vi "ExPhotometricsAsync.vi"() -> ()   [LabVIEW 2010]
panel:
  in  "Shutter end state":u32(ring)=1 items=["N/A", "No Change (keep cc and shutter as is)", "Halt (No Cont Clears)", "Halt Close shutter (No cont. clears)", "Clear (turn on cont clears)", "Clear and close shutter (cc on, shutter closed)", "Open shutter (no cont clears)", "Clear and open shutter (cc on, shutter open)", ""]
  in  "Shutter State":u32(ring)=1 items=["N/A", "Shutter always closed.", "Shutter Normal (open for expos/close for readout)", "Shutter opened begin acquisition sequence", "Shutter open prior-trigger"]
  in  "Trigger Edge":u32(ring)=1 items=["N/A", "Positive (leading) edge", "Negative (falling) edge"]
  in  "Timing Mode":u32(ring)=1
  in  "Exposure":dbl min=0.0 step=0.001 format="%.3f"
  in  "stop":bool
  in  "Store":bool
  out "error out":errorcluster
  in  "error in (no error)":errorcluster
  # "ExPhotometricsAsync:\nThis is a Full Frame Async example dessigned specificly for \nPhotometrics cameras. This should work with \nall camera systems. It requires a start for every frame \ncollected. Not all timing modes work for all cameras, also \nthe trigger edge only applies to Princeton Instrument \ncameras. Not all cameras have the ability to set the \ntemperature.\nPressing the stop button stops the example."
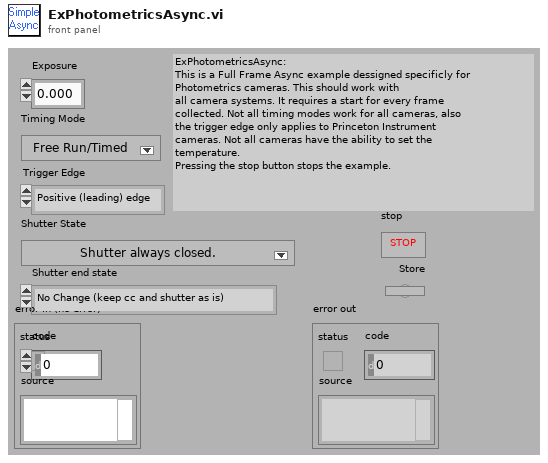
[diagram p1: front panel]
types:
  T1 = cluster{"Acquire mode \n3 is Async":i32, "Exposure":dbl, "Number of Images":i32, "Software Accums":i32}
  T2 = cluster{"Camera Handle":u32, "Pulser Handle":u32, "File Handle":u32, "Display Handle":u32, "Image Handle":u32}
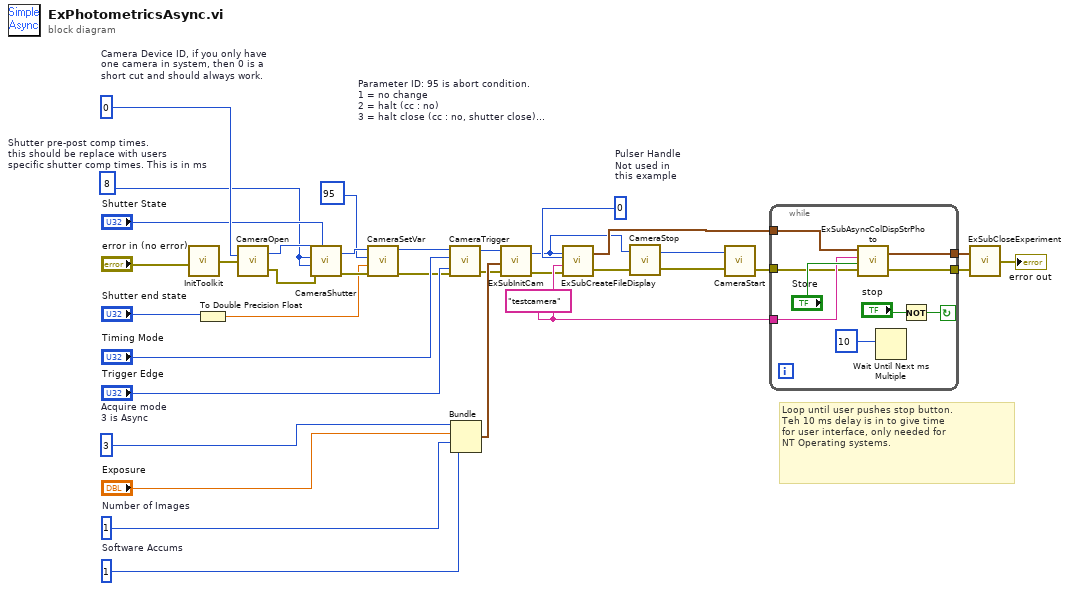
[diagram p0: block diagram]
diagram:
  w8 = 95  # Parameter ID: 95 is abort condition. 1 = no change 2 = halt (cc : no) 3 = halt close (cc : no, shutter close) 4 = clear (cc : yes) 5 = clear close (cc : yes, shutter close) 6 = open (cc : no, shutter open) 7 = clear open (cc : yes, shutter open)
  w13 = 8  # Shutter pre-post comp times. this should be replace with users  specific shutter comp times. This is in ms
  w21 = 0  # Camera Device ID, if you only have  one camera in system, then 0 is a  short cut and should always work.
  w28 = 0  # Pulser Handle Not used in  this example
  w33 = 1  # Number of Images
  w34 = 3  # Acquire mode  3 is Async
  w32 = 1  # Software Accums
  w35 = "testcamera"
  # "Loop until user pushes stop button.\nTeh 10 ms delay is in to give time \nfor user interface, only needed for \nNT Operating systems."
  n1 = call <userlib>:"InitToolkit.vi"("error in"="error in (no error)") -> ("error out"=w22:errorcluster)
  n2 = To Double Precision Float(number="Shutter end state") -> (double precision float=w6:dbl)
  n3 = call <userlib>:"CameraOpen.vi"("error in"=w22, "Camera Device ID"=w21) -> ("error out"=w14:errorcluster, "Camera Handle"=w15:u32)
  n4 = call <userlib>:"CameraShutter.vi"("Camera Handle"=w15, "Shutter Comp Time: Pre Open"=w13, "Shutter Comp Time: Post Open"=w13, "error in"=w14, "Shutter State"="Shutter State") -> ("Camera Handle"=w12:u32, "error out"=w11:errorcluster)
  n5 = call <userlib>:"CameraSetVar.vi"("error in"=w11, "Value"=w6, "Parameter ID"=w8, "Camera Handle"=w12) -> ("error out"=w10:errorcluster, "CameraHandle"=w9:u32)
  n6 = call <userlib>:"CameraTrigger.vi"("error in"=w10, "Trigger Edge"="Trigger Edge", "Timing Mode"="Timing Mode", "Camera Handle"=w9) -> ("error out"=w18:errorcluster, "Camera Handle"=w17:u32)
  n7 = Bundle("Acquire mode \n3 is Async"=w34, "Exposure"="Exposure", "Number of Images"=w33, "Software Accums"=w32) -> (w30:T1)  [unwired: 1 in]
  n8 = call "ExSubInitCam.vi"("error in (no error)"=w18, "Camera Information"=w30, "Camera Handle"=w17) -> ("error out"=w29:errorcluster, "Camera Handle"=w1:u32)
  n9 = call "ExSubCreateFileDisplay.vi"("error in (no error)"=w29, "File and Display Name"=w35, "Pulser Handle"=w28, "Camera Handle"=w1) -> ("error out"=w4:errorcluster, "Handles Out"=w5:T2)
  n10 = call <userlib>:"CameraStop.vi"("error in"=w4, "Camera Handle"=w1) -> ("error out"=w3:errorcluster, "Camera Handle"=w2:u32)
  n11 = call <userlib>:"CameraStart.vi"("error in"=w3, "Camera Handle"=w2) -> ("error out"=w27:errorcluster)  [unwired: 1 out]
  n12 = while {
    tunnel: w5 -> [w42]
    tunnel: w27 -> [w40]
    tunnel: w35 -> [w41]
    tunnel: [w38] -> w25
    tunnel: [w39] -> w26
    stop <- w37 continue-if-true
    n13 = call "ExSubAsyncColDispStrPhoto.vi"("error in (no error)"=w40, "Store Data"="Store", "Display Title"=w41, "Handle Cluster"=w42) -> ("error out"=w38:errorcluster, "Handle Cluster Out"=w39:T2)
    n14 = Wait Until Next ms Multiple(millisecond multiple=10) -> ()  [unwired: 1 out]
    n15 = Not(x="stop") -> (.not. x?=w37:bool)
  }
  n16 = call "ExSubCloseExperiment.vi"("error in (no error)"=w25, "Handles In"=w26) -> ("error out"=→"error out":errorcluster)
